vi "GET_issues_by_ids.vi"(8 "error in (no error)":errorcluster, 11 "REST Client in":refnum<class "REST Client.lvclass">) -> (0 "error out":errorcluster, 2 "local_issue":T1, 3 "REST Client out":refnum<class "REST Client.lvclass">)   [LabVIEW 2024]
uses:
  <vilib>/addons/_JKI.lib/REST Client/classes/REST Client/REST Client.lvclass
  definitions/local_issue.ctl
  definitions/comicvine_issue.generic_credit.ctl
  definitions/comicvine_issue.associated_image.ctl
  definitions/comicvine_issue.person_credit.ctl
  <vilib>/addons/_JKI.lib/REST Client/classes/REST Client/HTTP Header.ctl
  <vilib>/NI/Advanced HTTP Client/Header--Combo Box.ctl
  <vilib>/NI/Advanced HTTP Client/Session.lvclass
  <userlib>/_OpenG.lib/string/string.llb/openg_string.lvlib
  definitions/comicvine_issue.results.ctl
  definitions/comicvine_issue.ctl
  <vilib>/addons/_JKI.lib/Serialization/JSON/JKI JSON Serialization.lvlib
panel:
  out "resulting string":string
  in  "issue_ids":i32[](array[numeric])=array[22736 elements]
  out "Response body":string
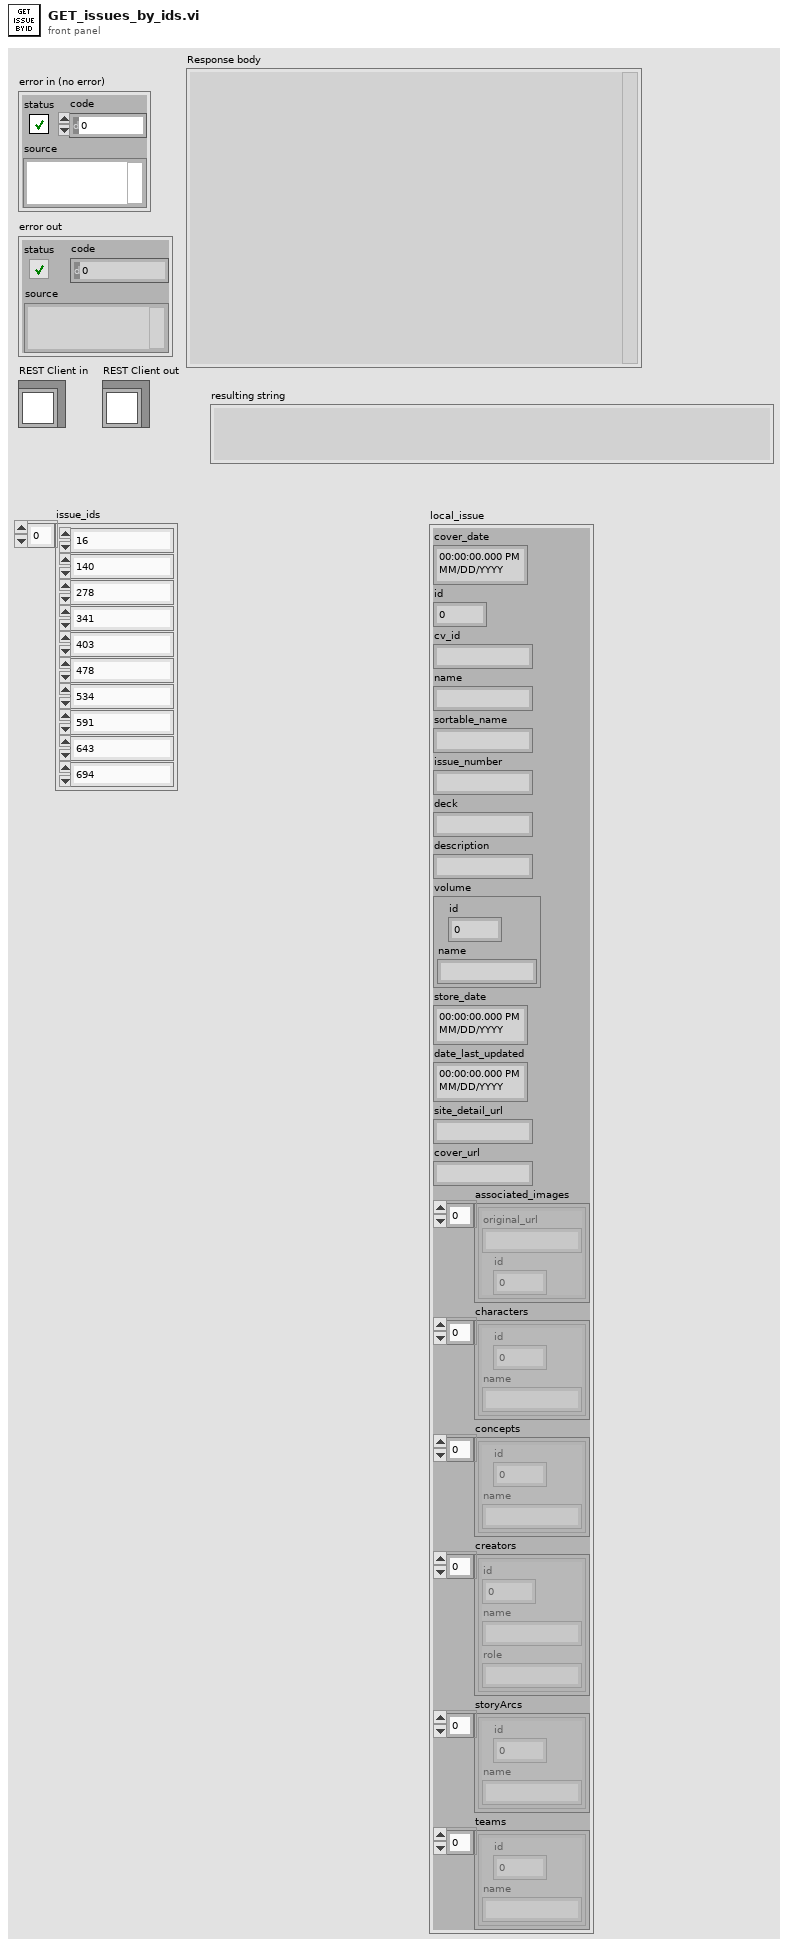
[diagram p1: front panel]
types:
  T1 = typedef "local_issue.ctl" = cluster{"cover_date":timestamp, "id":i32, "cv_id":string, "name":string, "sortable_name":string, "issue_number":string, "deck":string, "description":string, "volume":T2, "store_date":timestamp, "date_last_updated":timestamp, "site_detail_url":string, "cover_url":string, "associated_images":T3[], "characters":T2[], "concepts":T2[], "creators":T4[], "storyArcs":T2[], "teams":T2[]}
  T2 = typedef "comicvine_issue.generic_credit.ctl" = cluster{"id":i32, "name":string}
  T3 = typedef "comicvine_issue.associated_image.ctl" = cluster{"original_url":string, "id":i32}
  T4 = typedef "comicvine_issue.person_credit.ctl" = cluster{"id":i32, "name":string, "role":string}
  T5 = typedef "REST Client.lvlib/REST Client.lvclass/HTTP Header.ctl" = cluster{"header":T6, "value":string}
  T6 = typedef "lib_NI_Advanced HTTP Client.lvlib/Session.lvclass/Header--Combo Box.ctl" = string
  T7 = typedef "comicvine_issue.ctl" = cluster{"error":string, "limit":i32, "offset":i32, "number_of_page_results":i32, "number_of_total_results":i32, "status_code":i32, "results":T8}
  T8 = typedef "comicvine_issue.results.ctl" = cluster{"associated_images":T3[], "character_credits":T2[], "concept_credits":T2[], "cover_date":timestamp, "date_last_updated":timestamp, "deck":string, "description":string, "id":i32, "image":cluster{"original_url":string}, "issue_number":string, "name":string, "person_credits":T4[], "site_detail_url":string, "store_date":timestamp, "story_arc_credits":T2[], "team_credits":T2[], "volume":T2}
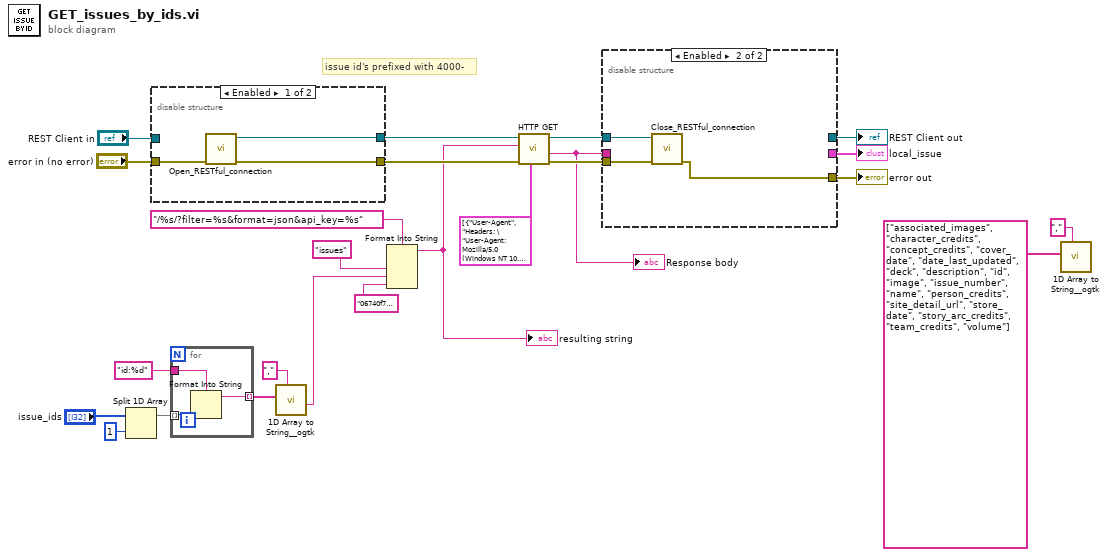
[diagram p0: block diagram]
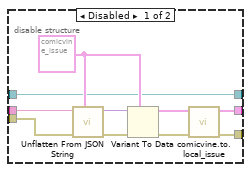
[diagram p2: hidden frame]
diagram:
  # "issue id's prefixed with 4000-"
  n1 = Split 1D Array(array="issue_ids", index=1) -> (first subarray=w6:i32[])  [unwired: 1 out]
  n2 = disable-structure shown="Enabled" {
    disable-tunnel: [w27 w28] -> w15
    disable-tunnel: [w26 w29] -> w14
    disable-tunnel: "error in (no error)" -> [w25 w29]
    disable-tunnel: "REST Client in" -> [_ w28]
    frame Enabled {
      n3 = call "Open_RESTful_connection.vi"("error in (no error)"=w25) -> ("error out"=w26:errorcluster, "REST Client out"=w27:refnum<class "REST Client.lvclass">)  [unwired: 9 in]
    }
    frame Disabled {
    }
  }
  n4 = for {
    tunnel: w6 -> [w31] mode=indexing
    tunnel: "id:%d" ("resource") -> [w32]
    tunnel: [w30] -> w4 mode=indexing
    n5 = Format Into String(format string=w32, w31) -> (resulting string=w30:string)  [unwired: 2 in, 1 out]
  }
  n6 = call <userlib>:"1D Array to String__ogtk.vi"("delimiter (Tab)"=",", "Array of Strings"=w4) -> ("delimited string"=w1:string)  [unwired: 9 in]
  n7 = Format Into String(format string="/%s/?filter=%s&format=json&api_key=%s", "issues" ("resource"), w1, "06740f73403e0b211d597c50ea94c7f16ea5e8ea") -> (resulting string=w2:string)  [unwired: 2 in, 1 out]
  "resulting string" <- w2
  n8 = call-dynamic "HTTP GET.vi"("request specific headers"=T5[] [{"header"="User-Agent", "value"="Headers: \"User-Agent: Mozilla/5.0 (Windows NT 10.0; Win64; x64) AppleWebKit/537.36 (KHTML, like Gecko) Chrome/91.0.4472.101 Safari/537.36\""}], "error in (no error)"=w14, "Path"=w2, "REST Client in"=w15) -> ("error out"=w24:errorcluster, "Response body"=w10:string, "REST Client out"=w11:refnum<class "REST Client.lvclass">)  [unwired: 2 in, 3 out]
  "Response body" <- w10
  n9 = disable-structure shown="Enabled" {
    disable-tunnel: w24 -> [w42 w44]
    disable-tunnel: w10 -> [w41 _]
    disable-tunnel: [w35 w43] -> w17
    disable-tunnel: [w34 _] -> w16
    disable-tunnel: w11 -> [w33 w45]
    disable-tunnel: [w33 _] -> w9
    frame Disabled {
      w38 = T7 {"error"="", "limit"=0, "offset"=0, "number_of_page_results"=0, "number_of_total_results"=0, "status_code"=0, "results"={"associated_images"=[], "character_credits"=[], "concept_credits"=[], "cover_date"=timestamp(0 s since 1904-01-01), "date_last_updated"=timestamp(0 s since 1904-01-01), "deck"="", "description"="", "id"=0, "image"={"original_url"=""}, "issue_number"="", "name"="", "person_credits"=[], "site_detail_url"="", "store_date"=timestamp(0 s since 1904-01-01), "story_arc_credits"=[], "team_credits"=[], "volume"={"id"=0, "name"=""}}} ("issue")
      n10 = call <vilib>:"Unflatten From JSON String.vi"("Type and Defaults"=w38, "error in (no error)"=w42, "JSON String"=w41) -> ("error out"=w40:errorcluster, "Variant"=w39:variant)  [unwired: 7 in]
      n11 = Variant To Data(error in=w40, type=w38, Variant=w39) -> (data=w37:T7, error out=w36:errorcluster)
      n12 = call "comicvine.to.local_issue.vi"("error in (no error)"=w36, "cv_issue"=w37) -> ("error out"=w35:errorcluster, "local_issue"=w34:T1)  [unwired: 8 in]
    }
    frame Enabled {
      n13 = call "Close_RESTful_connection.vi"("error in (no error)"=w44, "REST Client in"=w45) -> ("error out"=w43:errorcluster)  [unwired: 9 in]
    }
  }
  "error out" <- w17
  "REST Client out" <- w9
  "local_issue" <- w16
  n14 = call <userlib>:"1D Array to String__ogtk.vi"("delimiter (Tab)"=",", "Array of Strings"=string[] ["associated_images", "character_credits", "concept_credits", "cover_date", "date_last_updated", "deck", "description", "id", "image", "issue_number", "name", "person_credits", "site_detail_url", "store_date", "story_arc_credits", "team_credits", "volume"]) -> ()  [unwired: 9 in, 1 out]
